vi "WF3154 2Mod 4Ch Fault Injection.vi"(2 "Packet (1)":u64, 4 "WF3154 I/O":T1={"FIU CH0"="WF-3154 #1/CH0", "FIU CH1"="WF-3154 #1/CH1", "FIU CH2"="WF-3154 #1/CH2", "FIU CH3"="WF-3154 #1/CH3", "FIU CH4"="WF-3154 #2/CH0", "FIU CH5"="WF-3154 #2/CH1", "FIU CH6"="WF-3154 #2/CH2", "FIU CH7"="WF-3154 #2/CH3"}) -> ()   [LabVIEW 2010]
doc: "This VI should be used when having two units (8 channels)of WF-3154 when creating a custom FPGA for VeriStand.\nIt uses one (1) packet."
uses:
  <vilib>/eio/EIONode/EIONode.xnode
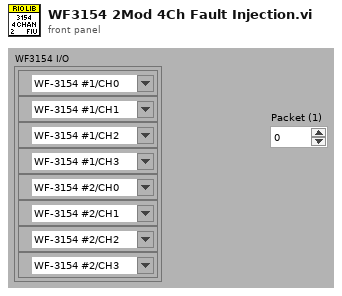
[diagram p1: front panel]
types:
  T1 = cluster{"FIU CH0":refnum<k21>, "FIU CH1":refnum<k21>, "FIU CH2":refnum<k21>, "FIU CH3":refnum<k21>, "FIU CH4":refnum<k21>, "FIU CH5":refnum<k21>, "FIU CH6":refnum<k21>, "FIU CH7":refnum<k21>}
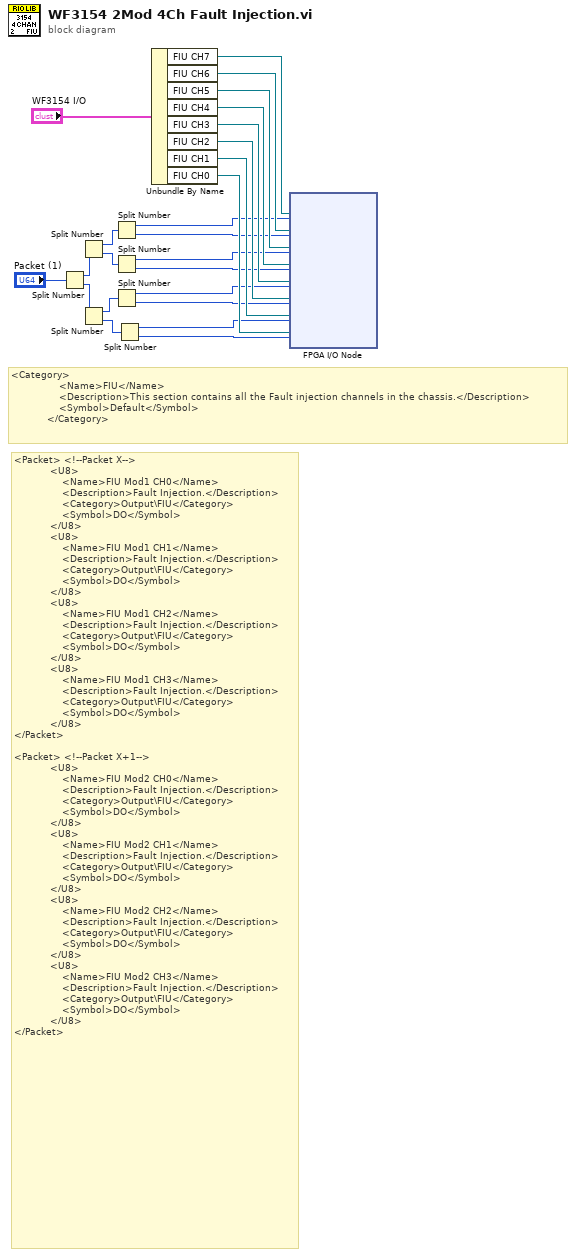
[diagram p0: block diagram]
diagram:
  # "<Packet>\t<!--Packet X-->\n            <U8>\n                <Name>FIU Mod1 CH0</Name>\n                <Description>Fault Injection.</Description>\n                <Category>Output\\FIU</Category>\n                <Symbol>DO</Symbol>\n            </U8>\n\t\t\t         <U8>\n                <Name>FIU Mod1 CH1</Name>\n                <Description>Fault Injection.</Description>\n                <Category>Output\\FIU</Category>\n                <Symbol>DO</Symbol>\n            </U8>\n\t\t\t         <U8>\n                <Name>FIU Mod1 CH2</Name>\n                <Description>Fault Injection.</Description>\n                <Category>Output\\FIU</Category>\n                <Symbol>DO</Symbol>\n            </U8>\n\t\t         \t<U8>\n                <Name>FIU Mod1 CH3</Name>\n                <Description>Fault Injection.</Description>\n                <Category>Output\\FIU</Category>\n                <Symbol>DO</Symbol>\n            </U8>\n</Packet>\n\n<Packet>\t<!--Packet X+1-->\n            <U8>\n                <Name>FIU Mod2 CH0</Name>\n                <Description>Fault Injection.</Description>\n                <Category>Output\\FIU</Category>\n                <Symbol>DO</Symbol>\n            </U8>\n\t\t\t         <U8>\n                <Name>FIU Mod2 CH1</Name>\n                <Description>Fault Injection.</Description>\n                <Category>Output\\FIU</Category>\n                <Symbol>DO</Symbol>\n            </U8>\n\t\t\t         <U8>\n                <Name>FIU Mod2 CH2</Name>\n                <Description>Fault Injection.</Description>\n                <Category>Output\\FIU</Category>\n                <Symbol>DO</Symbol>\n            </U8>\n\t\t\t         <U8>\n                <Name>FIU Mod2 CH3</Name>\n                <Description>Fault Injection.</Description>\n                <Category>Output\\FIU</Category>\n                <Symbol>DO</Symbol>\n            </U8>\n</Packet>"
  # "<Category>\n                <Name>FIU</Name>\n                <Description>This section contains all the Fault injection channels in the chassis.</Description>\n                <Symbol>Default</Symbol>\n            </Category>"
  n1 = Split Number(x="Packet (1)") -> (hi(x)=w14:u32, lo(x)=w15:u32)
  n2 = Split Number(x=w14) -> (hi(x)=w20:u16, lo(x)=w19:u16)
  n3 = Split Number(x=w15) -> (hi(x)=w16:u16, lo(x)=w17:u16)
  n4 = Split Number(x=w20) -> (hi(x)=w1:u8, lo(x)=w2:u8)
  n5 = Split Number(x=w19) -> (hi(x)=w4:u8, lo(x)=w3:u8)
  n6 = Split Number(x=w16) -> (hi(x)=w8:u8, lo(x)=w7:u8)
  n7 = Split Number(x=w17) -> (hi(x)=w6:u8, lo(x)=w5:u8)
  n8 = Unbundle By Name("WF3154 I/O") -> ("FIU CH7"=w23:refnum<k21>, "FIU CH6"=w22:refnum<k21>, "FIU CH5"=w21:refnum<k21>, "FIU CH4"=w18:refnum<k21>, "FIU CH3"=w12:refnum<k21>, "FIU CH2"=w11:refnum<k21>, "FIU CH1"=w10:refnum<k21>, "FIU CH0"=w9:refnum<k21>)
  n9 = xnode "FPGA I/O Node"("I/O Item"=w1, "FPGA I/O In"=w23, "I/O Item"=w2, "FPGA I/O In"=w22, "I/O Item"=w4, "FPGA I/O In"=w21, "I/O Item"=w3, "FPGA I/O In"=w18, "I/O Item"=w8, "FPGA I/O In"=w12, "I/O Item"=w7, "FPGA I/O In"=w11, "I/O Item"=w6, "FPGA I/O In"=w10, "I/O Item"=w5, "FPGA I/O In"=w9) -> ()  [unwired: 8 out]
